vi "UHR-Fleezers Control (host) - 11.8.vi"() -> ()   [LabVIEW 2014] (continued)
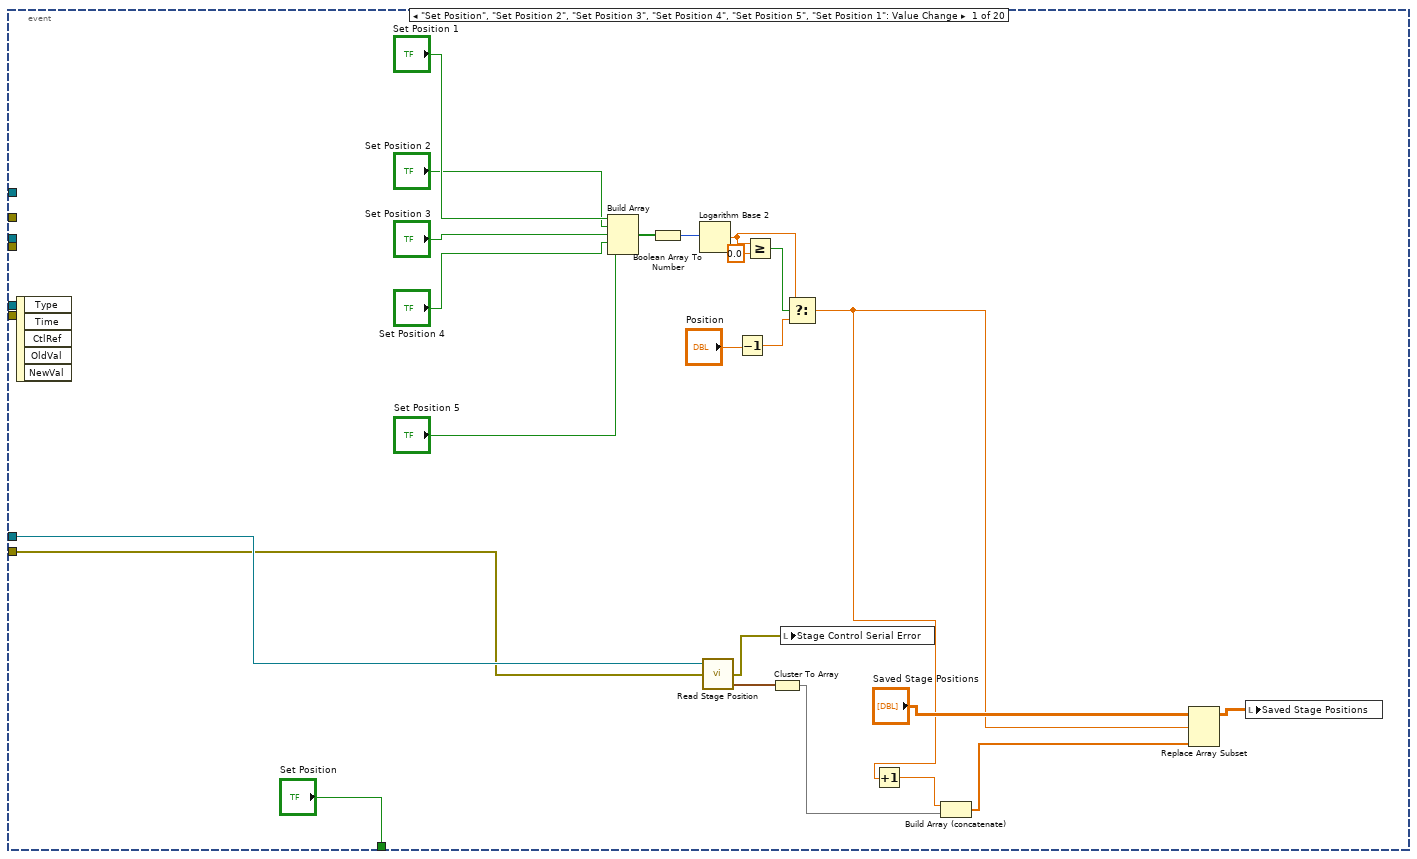
[diagram p2: hidden frame]
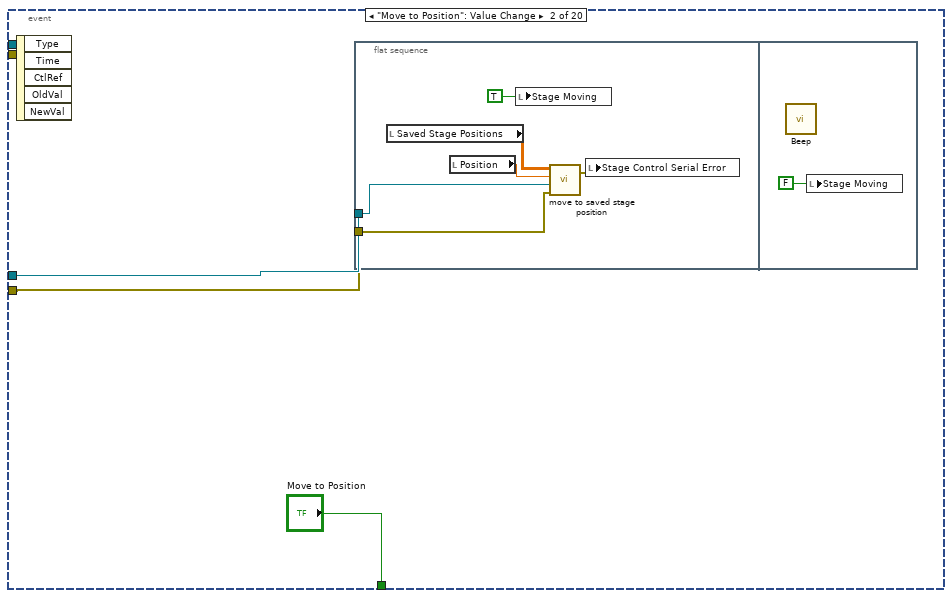
[diagram p3: hidden frame]
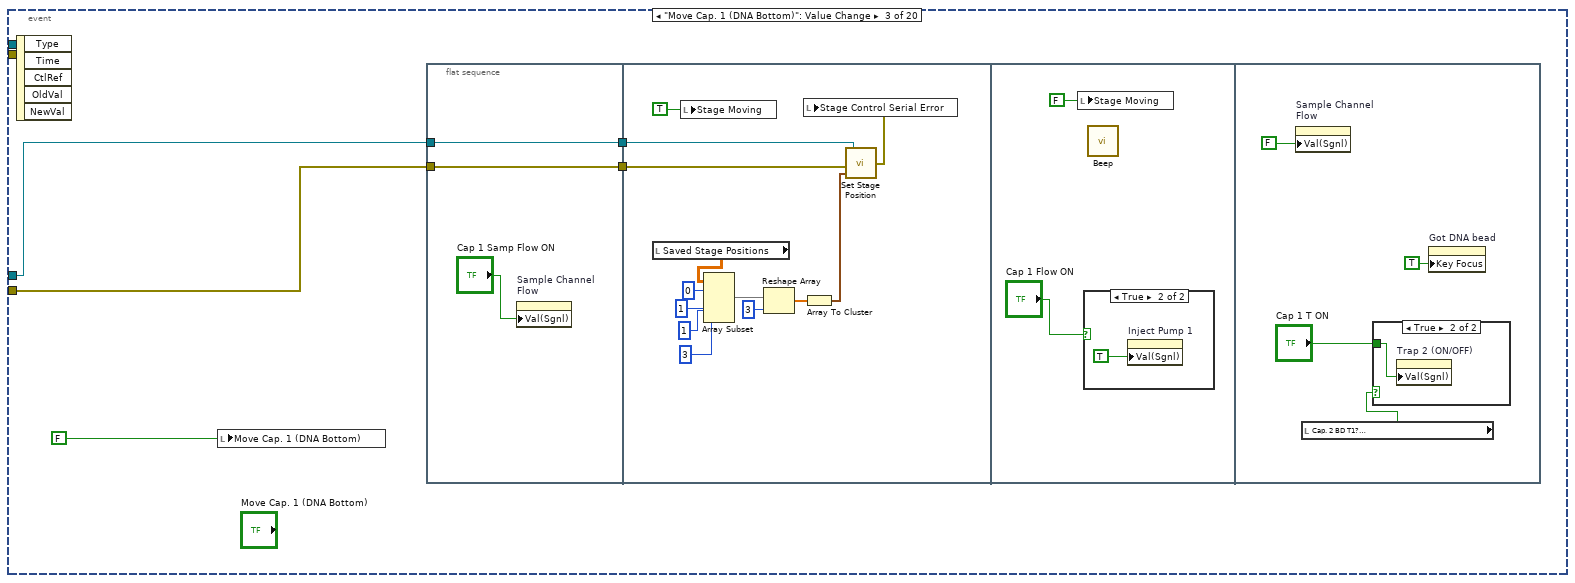
[diagram p4: hidden frame]
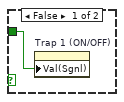
[diagram p6: hidden frame]
                n3338 = Subtract(x=w5153, y=w5152) -> (x-y=w5150:dbl)
                "Delta Fl. 1" <- w5150
                n3339 = Initialize Array(w5150, 1 ("dimension size")) -> (w5147:dbl[])
                n3340 = Initialize Array(w5119, 1 ("dimension size")) -> (w5124:dbl[])
                n3341 = feedback #42(w5147) -> (w5148:dbl[])
                n3342 = Build Array (concatenate)(w5148, w5147) -> (w5146:dbl[])
                n3343 = feedback #43(w5124) -> (w5125:dbl[])
                n3344 = Build Array (concatenate)(w5125, w5124) -> (w5123:dbl[])
                n3345 = feedback #44(w5107) -> (w5106:dbl[])
                n3346 = Build Array (concatenate)(w5106, w5107) -> (w5108:dbl[])
                n3347 = Select(t=w5107, s=w5109, f=w5108) -> (s? t:f=w5105:dbl[])
                "Saved trap pos" <- w5105
                n3348 = feedback-in #44(w5105) -> ()
                n3349 = Select(t=w5147, s=w5109, f=w5146) -> (s? t:f=w5122:dbl[])
                n3350 = feedback-in #42(w5122) -> ()
                n3351 = Select(t=w5124, s=w5109, f=w5123) -> (s? t:f=w5121:dbl[])
                n3352 = feedback-in #43(w5121) -> ()
                n3353 = Build Array(w5122, w5121) -> (→"Save APD Deriv":dbl[][])
              }
            }
            "Progress" <- w5088
            "Progress 2" <- w5088
          }
        }
      }
    }
    n3354 = Bundle By Name(cluster=w3682, "Green FB Ch 0"=w3681, "Green FB Ch 1"=w3680) -> (w3660:T48)
    "Green FB Signals (V)" <- w3660
    n3355 = Unbundle By Name(w3660) -> ("Green FB Ch 2"=→"Green FB Plot":dbl)
    n3356 = local read "wait to reset values"() -> (w3750:bool)
    n3357 = Not(x=w3748) -> (.not. x?=w3751:bool)
    n3358 = And(x=w3751, y=w3750) -> (x .and. y?=w3752:bool)
    n3359 = case "Part of MCL raster scanning: returns to initial positions after scan done" shown="True" w3752 {
      tunnel: w3469 -> [w4623 w4630]
      tunnel: [w4623 w4629] -> w3754
      tunnel: w3468 -> [w4622 w4628]
      tunnel: [w4622 w4627] -> w3749
      frame False {
      }
      frame True {
        w4638 = 10.0 ("y")
        w4637 = 32767.0 ("y")
        # "to return scan values\nafter a synchronous \nAOM scan"
        n3360 = local read "AO2"() -> (w4631:dbl)
        n3361 = local read "AO1"() -> (w4632:dbl)
        n3362 = local write "wait to reset values"(FALSE ("wait to reset values")) -> ()
        n3363 = Multiply(x=w4632, y=w4637) -> (x*y=w4634:dbl)
        n3364 = Multiply(x=w4631, y=w4637) -> (x*y=w4636:dbl)
        n3365 = Divide(x=w4634, y=w4638) -> (x/y=w4633:dbl)
        n3366 = Divide(x=w4636, y=w4638) -> (x/y=w4635:dbl)
        n3367 = To Word Integer(number=w4633) -> (16bit integer=w4639:i16)
        n3368 = To Word Integer(number=w4635) -> (16bit integer=w4640:i16)
        n3369 = local read "Total Counts (ticks)"() -> (w4624:u32)
        n3370 = xnode "Read/Write Control"("FPGA VI Reference In"=w4630, "error in"=w4628, "AO1"=w4639, "AO2"=w4640, "MCL count"=w4624) -> ("FPGA VI Reference Out"=w4629:T19, "error out"=w4627:errorcluster)
        n3371 = local read "Scan Range (V)\n(of steps)"() -> (w4625:dbl)
        n3372 = property on="Scan Range (V)\n(of steps)" class="DigNum (strict)"("Val(Sgnl)"=w4625) -> ()  [unwired: 2 in, 2 out]
      }
    }
    n3373 = node-c288() -> ()  [unwired: 2 out]
  }
  n3374 = VISA Close(VISA resource name=w99, error in (no error)=w98) -> (error out=w146:errorcluster)
  n3375 = call <vilib>:"Simple Error Handler.vi"("error in (no error)"=w146) -> ()  [unwired: 1 in, 8 out]
  n3376 = node-c288(w105) -> ()  [unwired: 1 out]
  n3377 = node-c288(w190) -> ()  [unwired: 1 out]
  n3378 = flat-sequence {
    tunnel: w282 -> [w5225]
    tunnel: w284 -> [w5226]
    tunnel: [w5224] -> w263
    tunnel: [w5223] -> w262
    tunnel: w246 -> [_]
    tunnel: w198 -> [_]
    tunnel: w111 -> [_]
    tunnel: w263 -> [w5227]
    tunnel: w262 -> [w5228]
    frame #0 {
      w5222 = FALSE ("AI to FIFO")
      n3379 = xnode "Read/Write Control"("FPGA VI Reference In"=w5226, "error in"=w5225, "AI to FIFO"=w5222, "APD to FIFO"=w5222) -> ("FPGA VI Reference Out"=w5224:T19, "error out"=w5223:errorcluster)
    }
    frame #1 {
      n3380 = xnode "Close FPGA VI Reference"("FPGA VI Reference In"=w5227, "error in"=w5228) -> ("error out"=→"error out":errorcluster)
    }
  }
